vi "nanocal -- nuclear schottky fit -- 2x2 -- V9.vi"() -> ()   [LabVIEW 2021] (continued)
1\" -> 0.000000000000   ,  \"mm2\" -> 0.000000000000   ,  \"mm3\" -> 0.000000000000   ,  \"T\" -> 1.120000000000   ,  \"B\" -> 2.000000000000   ,  \"θ\" -> 90.000000000000   ,  \"Reoff\" -> 0.000000000000   ,  \"Imoff\" -> 0.000000000000   ,  \"στ1\" -> 0.000000000000   ,  \"στS\" -> 0.000000000000   ,  \"στN\" -> 0.000000000000    |>   , \n\"IDS0590_220608_RAW_cal__ref_\" ->   <|    \"ζ\" -> 0.017825574653   ,  \"τ1\" -> 0.116468007826   ,  \"τS\" -> 0.043141778106   ,  \"τN\" -> 0.000373800852   ,  \"τC\" -> 0.002722368928   ,  \"κ0\" -> 0.000000010436   ,  \"mm1\" -> 0.000044937841   ,  \"mm2\" -> 0.046336871767   ,  \"mm3\" -> 0.117099836305   ,  \"T\" -> 1.600000000000   ,  \"B\" -> 2.000000000000   ,  \"θ\" -> 90.000000000000   ,  \"Reoff\" -> -510204.081632653076   ,  \"Imoff\" -> 0.000000000000   ,  \"στ1\" -> 0.011139723010   ,  \"στS\" -> 0.000337999811   ,  \"στN\" -> 0.000011692762    |>   , \n\"IDS0590_220608_RAW_cal__sam_\" ->   <|    \"ζ\" -> 0.000000000000   ,  \"τ1\" -> 0.000000000000   ,  \"τS\" -> 0.000000000000   ,  \"τN\" -> 0.000000000000   ,  \"τC\" -> 0.000000000000   ,  \"κ0\" -> 0.000000000000   ,  \"mm1\" -> 0.000000000000   ,  \"mm2\" -> 0.000000000000   ,  \"mm3\" -> 0.000000000000   ,  \"T\" -> 1.600000000000   ,  \"B\" -> 2.000000000000   ,  \"θ\" -> 90.000000000000   ,  \"Reoff\" -> 0.000000000000   ,  \"Imoff\" -> 0.000000000000   ,  \"στ1\" -> 0.000000000000   ,  \"στS\" -> 0.000000000000   ,  \"στN\" -> 0.000000000000    |>   , \n\"IDS0591_220608_RAW_cal__ref_\" ->   <|    \"ζ\" -> 0.018966449660   ,  \"τ1\" -> 0.110092167291   ,  \"τS\" -> 0.012256930668   ,  \"τN\" -> 0.000242942358   ,  \"τC\" -> 0.002442548821   ,  \"κ0\" -> 0.000000015655   ,  \"mm1\" -> 0.000038124511   ,  \"mm2\" -> 0.014855231202   ,  \"mm3\" -> 0.110378311637   ,  \"T\" -> 2.300000000000   ,  \"B\" -> 2.000000000000   ,  \"θ\" -> 90.000000000000   ,  \"Reoff\" -> -330612.244897959171   ,  \"Imoff\" -> 0.000000000000   ,  \"στ1\" -> 0.010082943855   ,  \"στS\" -> 0.000135571063   ,  \"στN\" -> 0.000004812408    |>   , \n\"IDS0591_220608_RAW_cal__sam_\" ->   <|    \"ζ\" -> 0.000000000000   ,  \"τ1\" -> 0.000000000000   ,  \"τS\" -> 0.000000000000   ,  \"τN\" -> 0.000000000000   ,  \"τC\" -> 0.000000000000   ,  \"κ0\" -> 0.000000000000   ,  \"mm1\" -> 0.000000000000   ,  \"mm2\" -> 0.000000000000   ,  \"mm3\" -> 0.000000000000   ,  \"T\" -> 2.300000000000   ,  \"B\" -> 2.000000000000   ,  \"θ\" -> 90.000000000000   ,  \"Reoff\" -> 0.000000000000   ,  \"Imoff\" -> 0.000000000000   ,  \"στ1\" -> 0.000000000000   ,  \"στS\" -> 0.000000000000   ,  \"στN\" -> 0.000000000000    |>   , \n\"IDS0592_220608_RAW_cal__ref_\" ->   <|    \"ζ\" -> 0.019357316755   ,  \"τ1\" -> 0.109232590741   ,  \"τS\" -> 0.009736709939   ,  \"τN\" -> 0.000148850192   ,  \"τC\" -> 0.002349823712   ,  \"κ0\" -> 0.000000022430   ,  \"mm1\" -> 0.000036187001   ,  \"mm2\" -> 0.012219724348   ,  \"mm3\" -> 0.109403421154   ,  \"T\" -> 3.100000000000   ,  \"B\" -> 2.000000000000   ,  \"θ\" -> 90.000000000000   ,  \"Reoff\" -> -232653.061224489822   ,  \"Imoff\" -> 0.000000000000   ,  \"στ1\" -> 0.008987310328   ,  \"στS\" -> 0.000109754464   ,  \"στN\" -> 0.000004448461    |>   , \n\"IDS0592_220608_RAW_cal__sam_\" ->   <|    \"ζ\" -> 0.000000000000   ,  \"τ1\" -> 0.000000000000   ,  \"τS\" -> 0.000000000000   ,  \"τN\" -> 0.000000000000   ,  \"τC\" -> 0.000000000000   ,  \"κ0\" -> 0.000000000000   ,  \"mm1\" -> 0.000000000000   ,  \"mm2\" -> 0.000000000000   ,  \"mm3\" -> 0.000000000000   ,  \"T\" -> 3.100000000000   ,  \"B\" -> 2.000000000000   ,  \"θ\" -> 90.000000000000   ,  \"Reoff\" -> 0.000000000000   ,  \"Imoff\" -> 0.000000000000   ,  \"στ1\" -> 0.000000000000   ,  \"στS\" -> 0.000000000000   ,  \"στN\" -> 0.000000000000    |>   , \n\"IDS0593_220608_RAW_cal__ref_\" ->   <|    \"ζ\" -> 0.022440001502   ,  \"τ1\" -> 0.108774382212   ,  \"τS\" -> 0.005986162529   ,  \"τN\" -> 0.000081229667   ,  \"τC\" -> 0.001771054543   ,  \"κ0\" -> 0.000000055356   ,  \"mm1\" -> 0.000030262826   ,  \"mm2\" -> 0.007854826642   ,  \"mm3\" -> 0.108863891772   ,  \"T\" -> 5.700000000000   ,  \"B\" -> 2.000000000000   ,  \"θ\" -> 90.000000000000   ,  \"Reoff\" -> -118367.346938775503   ,  \"Imoff\" -> 0.000000000000   ,  \"στ1\" -> 0.009498599420   ,  \"στS\" -> 0.000059156113   ,  \"στN\" -> 0.000001864029    |>   , \n\"IDS0593_220608_RAW_cal__sam_\" ->   <|    \"ζ\" -> 0.000000000000   ,  \"τ1\" -> 0.000000000000   ,  \"τS\" -> 0.000000000000   ,  \"τN\" -> 0.000000000000   ,  \"τC\" -> 0.000000000000   ,  \"κ0\" -> 0.000000000000   ,  \"mm1\" -> 0.000000000000   ,  \"mm2\" -> 0.000000000000   ,  \"mm3\" -> 0.000000000000   ,  \"T\" -> 5.700000000000   ,  \"B\" -> 2.000000000000   ,  \"θ\" -> 90.000000000000   ,  \"Reoff\" -> 0.000000000000   ,  \"Imoff\" -> 0.000000000000   ,  \"στ1\" -> 0.000000000000   ,  \"στS\" -> 0.000000000000   ,  \"στN\" -> 0.000000000000    |>   , \n\"IDS0595_220608_RAW_cal__ref_\" ->   <|    \"ζ\" -> 0.258873400405   ,  \"τ1\" -> 0.044703065528   ,  \"τS\" -> 0.045959272173   ,  \"τN\" -> 0.010257269472   ,  \"τC\" -> 0.000790030370   ,  \"κ0\" -> 0.000000000876   ,  \"mm1\" -> 0.000160711520   ,  \"mm2\" -> 0.030566838015   ,  \"mm3\" -> 0.085535055303   ,  \"T\" -> 0.200000000000   ,  \"B\" -> 4.000000000000   ,  \"θ\" -> 90.000000000000   ,  \"Reoff\" -> -50122448.979591846500   ,  \"Imoff\" -> 0.000000000000   ,  \"στ1\" -> 0.022832091218   ,  \"στS\" -> 0.001836443517   ,  \"στN\" -> 0.003113362841    |>   , \n\"IDS0595_220608_RAW_cal__sam_\" ->   <|    \"ζ\" -> 0.000000000000   ,  \"τ1\" -> 0.000000000000   ,  \"τS\" -> 0.000000000000   ,  \"τN\" -> 0.000000000000   ,  \"τC\" -> 0.000000000000   ,  \"κ0\" -> 0.000000000000   ,  \"mm1\" -> 0.000000000000   ,  \"mm2\" -> 0.000000000000   ,  \"mm3\" -> 0.000000000000   ,  \"T\" -> 0.200000000000   ,  \"B\" -> 4.000000000000   ,  \"θ\" -> 90.000000000000   ,  \"Reoff\" -> 0.000000000000   ,  \"Imoff\" -> 0.000000000000   ,  \"στ1\" -> 0.000000000000   ,  \"στS\" -> 0.000000000000   ,  \"στN\" -> 0.000000000000    |>   , \n\"IDS0596_220608_RAW_cal__ref_\" ->   <|    \"ζ\" -> 0.360293553844   ,  \"τ1\" -> 0.054491247205   ,  \"τS\" -> 0.052365925569   ,  \"τN\" -> 0.021163604976   ,  \"τC\" -> 0.000735569124   ,  \"κ0\" -> 0.000000000708   ,  \"mm1\" -> 0.000193352298   ,  \"mm2\" -> 0.031708785760   ,  \"mm3\" -> 0.123346424689   ,  \"T\" -> 0.170000000000   ,  \"B\" -> 4.000000000000   ,  \"θ\" -> 90.000000000000   ,  \"Reoff\" -> -91020408.163265347500   ,  \"Imoff\" -> 0.000000000000   ,  \"στ1\" -> 0.039757626567   ,  \"στS\" -> 0.004569334706   ,  \"στN\" -> 0.007867287880    |>   , \n\"IDS0596_220608_RAW_cal__sam_\" ->   <|    \"ζ\" -> 0.000000000000   ,  \"τ1\" -> 0.000000000000   ,  \"τS\" -> 0.000000000000   ,  \"τN\" -> 0.000000000000   ,  \"τC\" -> 0.000000000000   ,  \"κ0\" -> 0.000000000000   ,  \"mm1\" -> 0.000000000000   ,  \"mm2\" -> 0.000000000000   ,  \"mm3\" -> 0.000000000000   ,  \"T\" -> 0.170000000000   ,  \"B\" -> 4.000000000000   ,  \"θ\" -> 90.000000000000   ,  \"Reoff\" -> 0.000000000000   ,  \"Imoff\" -> 0.000000000000   ,  \"στ1\" -> 0.000000000000   ,  \"στS\" -> 0.000000000000   ,  \"στN\" -> 0.000000000000    |>   , \n\"IDS0597_220608_RAW_cal__ref_\" ->   <|    \"ζ\" -> 0.463165977160   ,  \"τ1\" -> 0.056305688672   ,  \"τS\" -> 0.058936067293   ,  \"τN\" -> 0.032266294348   ,  \"τC\" -> 0.000690215533   ,  \"κ0\" -> 0.000000000590   ,  \"mm1\" -> 0.000217293879   ,  \"mm2\" -> 0.030581784486   ,  \"mm3\" -> 0.159641018430   ,  \"T\" -> 0.150000000000   ,  \"B\" -> 4.000000000000   ,  \"θ\" -> 90.000000000000   ,  \"Reoff\" -> -129873469.387755096000   ,  \"Imoff\" -> 0.000000000000   ,  \"στ1\" -> 0.023207253822   ,  \"στS\" -> 0.004087293472   ,  \"στN\" -> 0.007020371426    |>   , \n\"IDS0597_220608_RAW_cal__sam_\" ->   <|    \"ζ\" -> 0.000000000000   ,  \"τ1\" -> 0.000000000000   ,  \"τS\" -> 0.000000000000   ,  \"τN\" -> 0.000000000000   ,  \"τC\" -> 0.000000000000   ,  \"κ0\" -> 0.000000000000   ,  \"mm1\" -> 0.000000000000   ,  \"mm2\" -> 0.000000000000   ,  \"mm3\" -> 0.000000000000   ,  \"T\" -> 0.150000000000   ,  \"B\" -> 4.000000000000   ,  \"θ\" -> 90.000000000000   ,  \"Reoff\" -> 0.000000000000   ,  \"Imoff\" -> 0.000000000000   ,  \"στ1\" -> 0.000000000000   ,  \"στS\" -> 0.000000000000   ,  \"στN\" -> 0.000000000000    |>   , \n\"IDS0598_220609_RAW_cal__ref_\" ->   <|    \"ζ\" -> 0.667698633058   ,  \"τ1\" -> 0.058414013789   ,  \"τS\" -> 0.079345994200   ,  \"τN\" -> 0.070623883647   ,  \"τC\" -> 0.000796244293   ,  \"κ0\" -> 0.000000000447   ,  \"mm1\" -> 0.000317638863   ,  \"mm2\" -> 0.027565245662   ,  \"mm3\" -> 0.281431933842   ,  \"T\" -> 0.120000000000   ,  \"B\" -> 4.000000000000   ,  \"θ\" -> 90.000000000000   ,  \"Reoff\" -> -199400000.000000000000   ,  \"Imoff\" -> 0.000000000000   ,  \"στ1\" -> 0.061256230703   ,  \"στS\" -> 0.021100595545   ,  \"στN\" -> 0.037759623008    |>   , \n\"IDS0598_220609_RAW_cal__sam_\" ->   <|    \"ζ\" -> 0.000000000000   ,  \"τ1\" -> 0.000000000000   ,  \"τS\" -> 0.000000000000   ,  \"τN\" -> 0.000000000000   ,  \"τC\" -> 0.000000000000   ,  \"κ0\" -> 0.000000000000   ,  \"mm1\" -> 0.000000000000   ,  \"mm2\" -> 0.000000000000   ,  \"mm3\" -> 0.000000000000   ,  \"T\" -> 0.120000000000   ,  \"B\" -> 4.000000000000   ,  \"θ\" -> 90.000000000000   ,  \"Reoff\" -> 0.000000000000   ,  \"Imoff\" -> 0.000000000000   ,  \"στ1\" -> 0.000000000000   ,  \"στS\" -> 0.000000000000   ,  \"στN\" -> 0.000000000000    |>   , \n\"IDS0599_220609_RAW_cal__ref_\" ->   <|    \"ζ\" -> 0.172195485890   ,  \"τ1\" -> 0.041384778581   ,  \"τS\" -> 0.038526635798   ,  \"τN\" -> 0.004361184391   ,  \"τC\" -> 0.000785294253   ,  \"κ0\" -> 0.000000001211   ,  \"mm1\" -> 0.000113668710   ,  \"mm2\" -> 0.030854392047   ,  \"mm3\" -> 0.061474921303   ,  \"T\" -> 0.250000000000   ,  \"B\" -> 4.000000000000   ,  \"θ\" -> 90.000000000000   ,  \"Reoff\" -> -31567346.938775509600   ,  \"Imoff\" -> 0.000000000000   ,  \"στ1\" -> 0.007771542596   ,  \"στS\" -> 0.000527239898   ,  \"στN\" -> 0.000989287072    |>   , \n\"IDS0599_220609_RAW_cal__sam_\" ->   <|    \"ζ\" -> 0.000000000000   ,  \"τ1\" -> 0.000000000000   ,  \"τS\" -> 0.000000000000   ,  \"τN\" -> 0.000000000000   ,  \"τC\" -> 0.000000000000   ,  \"κ0\" -> 0.000000000000   ,  \"mm1\" -> 0.000000000000   ,  \"mm2\" -> 0.000000000000   ,  \"mm3\" -> 0.000000000000   ,  \"T\" -> 0.250000000000   ,  \"B\" -> 4.000000000000   ,  \"θ\" -> 90.000000000000   ,  \"Reoff\" -> 0.000000000000   ,  \"Imoff\" -> 0.000000000000   ,  \"στ1\" -> 0.000000000000   ,  \"στS\" -> 0.000000000000   ,  \"στN\" -> 0.000000000000    |>   , \n\"IDS0601_220609_RAW_cal__ref_\" ->   <|    \"ζ\" -> 0.088588946696   ,  \"τ1\" -> 0.041065464736   ,  \"τS\" -> 0.032932718499   ,  \"τN\" -> 0.001668080480   ,  \"τC\" -> 0.000981218773   ,  \"κ0\" -> 0.000000001942   ,  \"mm1\" -> 0.000077888432   ,  \"mm2\" -> 0.031092575692   ,  \"mm3\" -> 0.048542266701   ,  \"T\" -> 0.360000000000   ,  \"B\" -> 4.000000000000   ,  \"θ\" -> 90.000000000000   ,  \"Reoff\" -> -11367346.938775509600   ,  \"Imoff\" -> 0.000000000000   ,  \"στ1\" -> 0.003759438303   ,  \"στS\" -> 0.000267670309   ,  \"στN\" -> 0.000061047491    |>   , \n\"IDS0601_220609_RAW_cal__sam_\" ->   <|    \"ζ\" -> 0.000000000000   ,  \"τ1\" -> 0.000000000000   ,  \"τS\" -> 0.000000000000   ,  \"τN\" -> 0.000000000000   ,  \"τC\" -> 0.000000000000   ,  \"κ0\" -> 0.000000000000   ,  \"mm1\" -> 0.000000000000   ,  \"mm2\" -> 0.000000000000   ,  \"mm3\" -> 0.000000000000   ,  \"T\" -> 0.360000000000   ,  \"B\" -> 4.000000000000   ,  \"θ\" -> 90.000000000000   ,  \"Reoff\" -> 0.000000000000   ,  \"Imoff\" -> 0.000000000000   ,  \"στ1\" -> 0.000000000000   ,  \"στS\" -> 0.000000000000   ,  \"στN\" -> 0.000000000000    |>   , \n\"IDS0602_220609_RAW_cal__ref_\" ->   <|    \"ζ\" -> 0.070839718876   ,  \"τ1\" -> 0.038371041474   ,  \"τS\" -> 0.031637984426   ,  \"τN\" -> 0.001186889357   ,  \"τC\" -> 0.001025755146   ,  \"κ0\" -> 0.000000002344   ,  \"mm1\" -> 0.000065987726   ,  \"mm2\" -> 0.030166305884   ,  \"mm3\" -> 0.044314681623   ,  \"T\" -> 0.420000000000   ,  \"B\" -> 4.000000000000   ,  \"θ\" -> 90.000000000000   ,  \"Reoff\" -> -8473469.387755101550   ,  \"Imoff\" -> 0.000000000000   ,  \"στ1\" -> 0.001572734023   ,  \"στS\" -> 0.000244025601   ,  \"στN\" -> 0.000010717849    |>   , \n\"IDS0602_220609_RAW_cal__sam_\" ->   <|    \"ζ\" -> 0.000000000000   ,  \"τ1\" -> 0.000000000000   ,  \"τS\" -> 0.000000000000   ,  \"τN\" -> 0.000000000000   ,  \"τC\" -> 0.000000000000   ,  \"κ0\" -> 0.000000000000   ,  \"mm1\" -> 0.000000000000   ,  \"mm2\" -> 0.000000000000   ,  \"mm3\" -> 0.000000000000   ,  \"T\" -> 0.420000000000   ,  \"B\" -> 4.000000000000   ,  \"θ\" -> 90.000000000000   ,  \"Reoff\" -> 0.000000000000   ,  \"Imoff\" -> 0.000000000000   ,  \"στ1\" -> 0.000000000000   ,  \"στS\" -> 0.000000000000   ,  \"στN\" -> 0.000000000000    |>   , \n\"IDS0603_220609_RAW_cal__ref_\" ->   <|    \"ζ\" -> 0.046492492626   ,  \"τ1\" -> 0.038232445790   ,  \"τS\" -> 0.031093656328   ,  \"τN\" -> 0.000672520001   ,  \"τC\" -> 0.001537595786   ,  \"κ0\" -> 0.000000003028   ,  \"mm1\" -> 0.000065353683   ,  \"mm2\" -> 0.030996834866   ,  \"mm3\" -> 0.041950918075   ,  \"T\" -> 0.520000000000   ,  \"B\" -> 4.000000000000   ,  \"θ\" -> 90.000000000000   ,  \"Reoff\" -> -3085714.285714285450   ,  \"Imoff\" -> 0.000000000000   ,  \"στ1\" -> 0.001914222591   ,  \"στS\" -> 0.000173880223   ,  \"στN\" -> 0.000009749430    |>   , \n\"IDS0603_220609_RAW_cal__sam_\" ->   <|    \"ζ\" -> 0.000000000000   ,  \"τ1\" -> 0.000000000000   ,  \"τS\" -> 0.000000000000   ,  \"τN\" -> 0.000000000000   ,  \"τC\" -> 0.000000000000   ,  \"κ0\" -> 0.000000000000   ,  \"mm1\" -> 0.000000000000   ,  \"mm2\" -> 0.000000000000   ,  \"mm3\" -> 0.000000000000   ,  \"T\" -> 0.520000000000   ,  \"B\" -> 4.000000000000   ,  \"θ\" -> 90.000000000000   ,  \"Reoff\" -> 0.000000000000   ,  \"Imoff\" -> 0.000000000000   ,  \"στ1\" -> 0.000000000000   ,  \"στS\" -> 0.000000000000   ,  \"στN\" -> 0.000000000000    |>   , \n\"IDS0604_220609_RAW_cal__ref_\" ->   <|    \"ζ\" -> 0.038076441388   ,  \"τ1\" -> 0.037827631760   ,  \"τS\" -> 0.031677046924   ,  \"τN\" -> 0.000456015371   ,  \"τC\" -> 0.001552950065   ,  \"κ0\" -> 0.000000003729   ,  \"mm1\" -> 0.000054479261   ,  \"mm2\" -> 0.031856398472   ,  \"mm3\" -> 0.040826279050   ,  \"T\" -> 0.620000000000   ,  \"B\" -> 4.000000000000   ,  \"θ\" -> 90.000000000000   ,  \"Reoff\" -> -2502040.816326530650   ,  \"Imoff\" -> 0.000000000000   ,  \"στ1\" -> 0.001808471812   ,  \"στS\" -> 0.000207619665   ,  \"στN\" -> 0.000014710860    |>   , \n\"IDS0604_220609_RAW_cal__sam_\" ->   <|    \"ζ\" -> 0.000000000000   ,  \"τ1\" -> 0.000000000000   ,  \"τS\" -> 0.000000000000   ,  \"τN\" -> 0.000000000000   ,  \"τC\" -> 0.000000000000   ,  \"κ0\" -> 0.000000000000   ,  \"mm1\" -> 0.000000000000   ,  \"mm2\" -> 0.000000000000   ,  \"mm3\" -> 0.000000000000   ,  \"T\" -> 0.620000000000   ,  \"B\" -> 4.000000000000   ,  \"θ\" -> 90.000000000000   ,  \"Reoff\" -> 0.000000000000   ,  \"Imoff\" -> 0.000000000000   ,  \"στ1\" -> 0.000000000000   ,  \"στS\" -> 0.000000000000   ,  \"στN\" -> 0.000000000000    |>   , \n\"IDS0605_220609_RAW_cal__ref_\" ->   <|    \"ζ\" -> 0.029084199331   ,  \"τ1\" -> 0.037802339111   ,  \"τS\" -> 0.034441444992   ,  \"τN\" -> 0.000221453940   ,  \"τC\" -> 0.001674221350   ,  \"κ0\" -> 0.000000005054   ,  \"mm1\" -> 0.000045238028   ,  \"mm2\" -> 0.034605412143   ,  \"mm3\" -> 0.040496951884   ,  \"T\" -> 0.820000000000   ,  \"B\" -> 4.000000000000   ,  \"θ\" -> 90.000000000000   ,  \"Reoff\" -> -1648979.591836734680   ,  \"Imoff\" -> 0.000000000000   ,  \"στ1\" -> 0.004366885644   ,  \"στS\" -> 0.000226589736   ,  \"στN\" -> 0.000007619141    |>   , \n\"IDS0605_220609_RAW_cal__sam_\" ->   <|    \"ζ\" -> 0.000000000000   ,  \"τ1\" -> 0.000000000000   ,  \"τS\" -> 0.000000000000   ,  \"τN\" -> 0.000000000000   ,  \"τC\" -> 0.000000000000   ,  \"κ0\" -> 0.000000000000   ,  \"mm1\" -> 0.000000000000   ,  \"mm2\" -> 0.000000000000   ,  \"mm3\" -> 0.000000000000   ,  \"T\" -> 0.820000000000   ,  \"B\" -> 4.000000000000   ,  \"θ\" -> 90.000000000000   ,  \"Reoff\" -> 0.000000000000   ,  \"Imoff\" -> 0.000000000000   ,  \"στ1\" -> 0.000000000000   ,  \"στS\" -> 0.000000000000   ,  \"στN\" -> 0.000000000000    |>   , \n\"IDS0606_220609_RAW_cal__ref_\" ->   <|    \"ζ\" -> 0.021888227668   ,  \"τ1\" -> 0.037829739612   ,  \"τS\" -> 0.039149374988   ,  \"τN\" -> 0.000098261842   ,  \"τC\" -> 0.001756976577   ,  \"κ0\" -> 0.000000007009   ,  \"mm1\" -> 0.000036081312   ,  \"mm2\" -> 0.037036868509   ,  \"mm3\" -> 0.042620464409   ,  \"T\" -> 1.100000000000   ,  \"B\" -> 4.000000000000   ,  \"θ\" -> 90.000000000000   ,  \"Reoff\" -> -840816.326530613004   ,  \"Imoff\" -> 0.000000000000   ,  \"στ1\" -> 0.002337246267   ,  \"στS\" -> 0.000239648135   ,  \"στN\" -> 0.000002696186    |>   , \n\"IDS0606_220609_RAW_cal__sam_\" ->   <|    \"ζ\" -> 0.000000000000   ,  \"τ1\" -> 0.000000000000   ,  \"τS\" -> 0.000000000000   ,  \"τN\" -> 0.000000000000   ,  \"τC\" -> 0.000000000000   ,  \"κ0\" -> 0.000000000000   ,  \"mm1\" -> 0.000000000000   ,  \"mm2\" -> 0.000000000000   ,  \"mm3\" -> 0.000000000000   ,  \"T\" -> 1.100000000000   ,  \"B\" -> 4.000000000000   ,  \"θ\" -> 90.000000000000   ,  \"Reoff\" -> 0.000000000000   ,  \"Imoff\" -> 0.000000000000   ,  \"στ1\" -> 0.000000000000   ,  \"στS\" -> 0.000000000000   ,  \"στN\" -> 0.000000000000    |>   , \n\"IDS0607_220609_RAW_cal__ref_\" ->   <|    \"ζ\" -> 0.018621761780   ,  \"τ1\" -> 0.037381709477   ,  \"τS\" -> 0.015442772270   ,  \"τN\" -> 0.000037477448   ,  \"τC\" -> 0.001928945161   ,  \"κ0\" -> 0.000000010412   ,  \"mm1\" -> 0.000031467858   ,  \"mm2\" -> 0.017593885804   ,  \"mm3\" -> 0.037453820216   ,  \"T\" -> 1.600000000000   ,  \"B\" -> 4.000000000000   ,  \"θ\" -> 90.000000000000   ,  \"Reoff\" -> -583673.469387755030   ,  \"Imoff\" -> 0.000000000000   ,  \"στ1\" -> 0.004296807814   ,  \"στS\" -> 0.000140639084   ,  \"στN\" -> 0.000001749476    |>   , \n\"IDS0607_220609_RAW_cal__sam_\" ->   <|    \"ζ\" -> 0.000000000000   ,  \"τ1\" -> 0.000000000000   ,  \"τS\" -> 0.000000000000   ,  \"τN\" -> 0.000000000000   ,  \"τC\" -> 0.000000000000   ,  \"κ0\" -> 0.000000000000   ,  \"mm1\" -> 0.000000000000   ,  \"mm2\" -> 0.000000000000   ,  \"mm3\" -> 0.000000000000   ,  \"T\" -> 1.600000000000   ,  \"B\" -> 4.000000000000   ,  \"θ\" -> 90.000000000000   ,  \"Reoff\" -> 0.000000000000   ,  \"Imoff\" -> 0.000000000000   ,  \"στ1\" -> 0.000000000000   ,  \"στS\" -> 0.000000000000   ,  \"στN\" -> 0.000000000000    |>   , \n\"IDS0608_220610_RAW_cal__ref_\" ->   <|    \"ζ\" -> 0.016544796602   ,  \"τ1\" -> 0.037383789571   ,  \"τS\" -> 0.013791768179   ,  \"τN\" -> 0.000022452051   ,  \"τC\" -> 0.002003011160   ,  \"κ0\" -> 0.000000012629   ,  \"mm1\" -> 0.000028575716   ,  \"mm2\" -> 0.015977354879   ,  \"mm3\" -> 0.037423643830   ,  \"T\" -> 1.900000000000   ,  \"B\" -> 4.000000000000   ,  \"θ\" -> 90.000000000000   ,  \"Reoff\" -> -306122.448979591834   ,  \"Imoff\" -> 0.000000000000   ,  \"στ1\" -> 0.018453773805   ,  \"στS\" -> 0.003656712594   ,  \"στN\" -> 0.000009862061    |>   , \n\"IDS0608_220610_RAW_cal__sam_\" ->   <|    \"ζ\" -> 0.000000000000   ,  \"τ1\" -> 0.000000000000   ,  \"τS\" -> 0.000000000000   ,  \"τN\" -> 0.000000000000   ,  \"τC\" -> 0.000000000000   ,  \"κ0\" -> 0.000000000000   ,  \"mm1\" -> 0.000000000000   ,  \"mm2\" -> 0.000000000000   ,  \"mm3\" -> 0.000000000000   ,  \"T\" -> 1.900000000000   ,  \"B\" -> 4.000000000000   ,  \"θ\" -> 90.000000000000   ,  \"Reoff\" -> 0.000000000000   ,  \"Imoff\" -> 0.000000000000   ,  \"στ1\" -> 0.000000000000   ,  \"στS\" -> 0.000000000000   ,  \"στN\" -> 0.000000000000    |>   , \n\"IDS0609_220610_RAW_cal__ref_\" ->   <|    \"ζ\" -> 0.016105107000   ,  \"τ1\" -> 0.037302695889   ,  \"τS\" -> 0.009839075109   ,  \"τN\" -> 0.000006613992   ,  \"τC\" -> 0.002285007383   ,  \"κ0\" -> 0.000000022392   ,  \"mm1\" -> 0.000029550397   ,  \"mm2\" -> 0.012249707235   ,  \"mm3\" -> 0.037312700617   ,  \"T\" -> 3.100000000000   ,  \"B\" -> 4.000000000000   ,  \"θ\" -> 90.000000000000   ,  \"Reoff\" -> -175510.204081632662   ,  \"Imoff\" -> 0.000000000000   ,  \"στ1\" -> 0.000595847504   ,  \"στS\" -> 0.000046124245   ,  \"στN\" -> 0.000000091796    |>   , \n\"IDS0609_220610_RAW_cal__sam_\" ->   <|    \"ζ\" -> 0.000000000000   ,  \"τ1\" -> 0.000000000000   ,  \"τS\" -> 0.000000000000   ,  \"τN\" -> 0.000000000000   ,  \"τC\" -> 0.000000000000   ,  \"κ0\" -> 0.000000000000   ,  \"mm1\" -> 0.000000000000   ,  \"mm2\" -> 0.000000000000   ,  \"mm3\" -> 0.000000000000   ,  \"T\" -> 3.100000000000   ,  \"B\" -> 4.000000000000   ,  \"θ\" -> 90.000000000000   ,  \"Reoff\" -> 0.000000000000   ,  \"Imoff\" -> 0.000000000000   ,  \"στ1\" -> 0.000000000000   ,  \"στS\" -> 0.000000000000   ,  \"στN\" -> 0.000000000000    |>   , \n\"IDS0610_220610_RAW_cal__ref_\" ->   <|    \"ζ\" -> 0.017289416692   ,  \"τ1\" -> 0.037297104830   ,  \"τS\" -> 0.006044321671   ,  \"τN\" -> 0.000001504072   ,  \"τC\" -> 0.001946264025   ,  \"κ0\" -> 0.000000055145   ,  \"mm1\" -> 0.000025203584   ,  \"mm2\" -> 0.008069462881   ,  \"mm3\" -> 0.037299056933   ,  \"T\" -> 5.700000000000   ,  \"B\" -> 4.000000000000   ,  \"θ\" -> 90.000000000000   ,  \"Reoff\" -> -61224.489795918343   ,  \"Imoff\" -> 0.000000000000   ,  \"στ1\" -> 0.009662236305   ,  \"στS\" -> 0.002526126048   ,  \"στN\" -> 0.000001649991    |>   , \n\"IDS0610_220610_RAW_cal__sam_\" ->   <|    \"ζ\" -> 0.000000000000   ,  \"τ1\" -> 0.000000000000   ,  \"τS\" -> 0.000000000000   ,  \"τN\" -> 0.000000000000   ,  \"τC\" -> 0.000000000000   ,  \"κ0\" -> 0.000000000000   ,  \"mm1\" -> 0.000000000000   ,  \"mm2\" -> 0.000000000000   ,  \"mm3\" -> 0.000000000000   ,  \"T\" -> 5.700000000000   ,  \"B\" -> 4.000000000000   ,  \"θ\" -> 90.000000000000   ,  \"Reoff\" -> 0.000000000000   ,  \"Imoff\" -> 0.000000000000   ,  \"στ1\" -> 0.000000000000   ,  \"στS\" -> 0.000000000000   ,  \"στN\" -> 0.000000000000    |>   , \n\"IDS0612_220610_RAW_cal__ref_\" ->   <|    \"ζ\" -> 0.027806171987   ,  \"τ1\" -> 0.017638558844   ,  \"τS\" -> 0.022454693159   ,  \"τN\" -> 0.000230606872   ,  \"τC\" -> 0.002790453039   ,  \"κ0\" -> 0.000000005094   ,  \"mm1\" -> 0.000067525510   ,  \"mm2\" -> 0.017167524250   ,  \"mm3\" -> 0.026510053509   ,  \"T\" -> 0.820000000000   ,  \"B\" -> 5.000000000000   ,  \"θ\" -> 90.000000000000   ,  \"Reoff\" -> -885714.285714285680   ,  \"Imoff\" -> 0.000000000000   ,  \"στ1\" -> 0.001146653541   ,  \"στS\" -> 0.000179915023   ,  \"στN\" -> 0.000004482288    |>   , \n\"IDS0612_220610_RAW_cal__sam_\" ->   <|    \"ζ\" -> 0.000000000000   ,  \"τ1\" -> 0.000000000000   ,  \"τS\" -> 0.000000000000   ,  \"τN\" -> 0.000000000000   ,  \"τC\" -> 0.000000000000   ,  \"κ0\" -> 0.000000000000   ,  \"mm1\" -> 0.000000000000   ,  \"mm2\" -> 0.000000000000   ,  \"mm3\" -> 0.000000000000   ,  \"T\" -> 0.820000000000   ,  \"B\" -> 5.000000000000   ,  \"θ\" -> 90.000000000000   ,  \"Reoff\" -> 0.000000000000   ,  \"Imoff\" -> 0.000000000000   ,  \"στ1\" -> 0.000000000000   ,  \"στS\" -> 0.000000000000   ,  \"στN\" -> 0.000000000000    |>   , \n\"IDS0613_220610_RAW_cal__ref_\" ->   <|    \"ζ\" -> 0.023917075048   ,  \"τ1\" -> 0.017613265802   ,  \"τS\" -> 0.018183300032   ,  \"τN\" -> 0.000148874581   ,  \"τC\" -> 0.002629507092   ,  \"κ0\" -> 0.000000007146   ,  \"mm1\" -> 0.000053956796   ,  \"mm2\" -> 0.016996296873   ,  \"mm3\" -> 0.021963145834   ,  \"T\" -> 1.120000000000   ,  \"B\" -> 5.000000000000   ,  \"θ\" -> 90.000000000000   ,  \"Reoff\" -> -877551.020408163311   ,  \"Imoff\" -> 0.000000000000   ,  \"στ1\" -> 0.001189746119   ,  \"στS\" -> 0.000158276904   ,  \"στN\" -> 0.000002453686    |>   , \n\"IDS0613_220610_RAW_cal__sam_\" ->   <|    \"ζ\" -> 0.000000000000   ,  \"τ1\" -> 0.000000000000   ,  \"τS\" -> 0.000000000000   ,  \"τN\" -> 0.000000000000   ,  \"τC\" -> 0.000000000000   ,  \"κ0\" -> 0.000000000000   ,  \"mm1\" -> 0.000000000000   ,  \"mm2\" -> 0.000000000000   ,  \"mm3\" -> 0.000000000000   ,  \"T\" -> 1.120000000000   ,  \"B\" -> 5.000000000000   ,  \"θ\" -> 90.000000000000   ,  \"Reoff\" -> 0.000000000000   ,  \"Imoff\" -> 0.000000000000   ,  \"στ1\" -> 0.000000000000   ,  \"στS\" -> 0.000000000000   ,  \"στN\" -> 0.000000000000    |>   , \n\"IDS0614_220610_RAW_cal__ref_\" ->   <|    \"ζ\" -> 0.017909358082   ,  \"τ1\" -> 0.017480687226   ,  \"τS\" -> 0.012860329043   ,  \"τN\" -> 0.000077799463   ,  \"τC\" -> 0.003015067786   ,  \"κ0\" -> 0.000000012573   ,  \"mm1\" -> 0.000043232989   ,  \"mm2\" -> 0.015457741040   ,  \"mm3\" -> 0.018164623065   ,  \"T\" -> 1.900000000000   ,  \"B\" -> 5.000000000000   ,  \"θ\" -> 90.000000000000   ,  \"Reoff\" -> -330612.244897959171   ,  \"Imoff\" -> 0.000000000000   ,  \"στ1\" -> 0.000912905894   ,  \"στS\" -> 0.000088716304   ,  \"στN\" -> 0.000002113548    |>   , \n\"IDS0614_220610_RAW_cal__sam_\" ->   <|    \"ζ\" -> 0.000000000000   ,  \"τ1\" -> 0.000000000000   ,  \"τS\" -> 0.000000000000   ,  \"τN\" -> 0.000000000000   ,  \"τC\" -> 0.000000000000   ,  \"κ0\" -> 0.000000000000   ,  \"mm1\" -> 0.000000000000   ,  \"mm2\" -> 0.000000000000   ,  \"mm3\" -> 0.000000000000   ,  \"T\" -> 1.900000000000   ,  \"B\" -> 5.000000000000   ,  \"θ\" -> 90.000000000000   ,  \"Reoff\" -> 0.000000000000   ,  \"Imoff\" -> 0.000000000000   ,  \"στ1\" -> 0.000000000000   ,  \"στS\" -> 0.000000000000   ,  \"στN\" -> 0.000000000000    |>   , \n\"IDS0615_220610_RAW_cal__ref_\" ->   <|    \"ζ\" -> 0.018184973350   ,  \"τ1\" -> 0.017408880913   ,  \"τS\" -> 0.009354983655   ,  \"τN\" -> 0.000026355523   ,  \"τC\" -> 0.002778499813   ,  \"κ0\" -> 0.000000022360   ,  \"mm1\" -> 0.000038538571   ,  \"mm2\" -> 0.012202232609   ,  \"mm3\" -> 0.017498548126   ,  \"T\" -> 3.100000000000   ,  \"B\" -> 5.000000000000   ,  \"θ\" -> 90.000000000000   ,  \"Reoff\" -> -191836.734693877515   ,  \"Imoff\" -> 0.000000000000   ,  \"στ1\" -> 0.001312365409   ,  \"στS\" -> 0.000063057161   ,  \"στN\" -> 0.000000988894    |>   , \n\"IDS0615_220610_RAW_cal__sam_\" ->   <|    \"ζ\" -> 0.000000000000   ,  \"τ1\" -> 0.000000000000   ,  \"τS\" -> 0.000000000000   ,  \"τN\" -> 0.000000000000   ,  \"τC\" -> 0.000000000000   ,  \"κ0\" -> 0.000000000000   ,  \"mm1\" -> 0.000000000000   ,  \"mm2\" -> 0.000000000000   ,  \"mm3\" -> 0.000000000000   ,  \"T\" -> 3.100000000000   ,  \"B\" -> 5.000000000000   ,  \"θ\" -> 90.000000000000   ,  \"Reoff\" -> 0.000000000000   ,  \"Imoff\" -> 0.000000000000   ,  \"στ1\" -> 0.000000000000   ,  \"στS\" -> 0.000000000000   ,  \"στN\" -> 0.000000000000    |>   , \n\"IDS0616_220610_RAW_cal__ref_\" ->   <|    \"ζ\" -> 0.021580744060   ,  \"τ1\" -> 0.018863304594   ,  \"τS\" -> 0.006040479317   ,  \"τN\" -> 0.000014968890   ,  \"τC\" -> 0.001981910818   ,  \"κ0\" -> 0.000000054950   ,  \"mm1\" -> 0.000031813796   ,  \"mm2\" -> 0.008109417181   ,  \"mm3\" -> 0.018890113720   ,  \"T\" -> 5.700000000000   ,  \"B\" -> 5.000000000000   ,  \"θ\" -> 90.000000000000   ,  \"Reoff\" -> -102040.816326530650   ,  \"Imoff\" -> 0.000000000000   ,  \"στ1\" -> 0.003832459400   ,  \"στS\" -> 0.000063285444   ,  \"στN\" -> 0.000001437164    |>   , \n\"IDS0616_220610_RAW_cal__sam_\" ->   <|    \"ζ\" -> 0.000000000000   ,  \"τ1\" -> 0.000000000000   ,  \"τS\" -> 0.000000000000   ,  \"τN\" -> 0.000000000000   ,  \"τC\" -> 0.000000000000   ,  \"κ0\" -> 0.000000000000   ,  \"mm1\" -> 0.000000000000   ,  \"mm2\" -> 0.000000000000   ,  \"mm3\" -> 0.000000000000   ,  \"T\" -> 5.700000000000   ,  \"B\" -> 5.000000000000   ,  \"θ\" -> 90.000000000000   ,  \"Reoff\" -> 0.000000000000   ,  \"Imoff\" -> 0.000000000000   ,  \"στ1\" -> 0.000000000000   ,  \"στS\" -> 0.000000000000   ,  \"στN\" -> 0.000000000000    |>   , \n\"IDS0618_220610_RAW_cal__ref_\" ->   <|    \"ζ\" -> 0.038971550776   ,  \"τ1\" -> 0.018146117143   ,  \"τS\" -> 0.027126639064   ,  \"τN\" -> 0.001095165707   ,  \"τC\" -> 0.001889759396   ,  \"κ0\" -> 0.000000003734   ,  \"mm1\" -> 0.000066576943   ,  \"mm2\" -> 0.016715518022   ,  \"mm3\" -> 0.032575433843   ,  \"T\" -> 0.620000000000   ,  \"B\" -> 8.000000000000   ,  \"θ\" -> 90.000000000000   ,  \"Reoff\" -> -2648979.591836734680   ,  \"Imoff\" -> 0.000000000000   ,  \"στ1\" -> 0.003517417724   ,  \"στS\" -> 0.000462948011   ,  \"στN\" -> 0.000116737620    |>   , \n\"IDS0618_220610_RAW_cal__sam_\" ->   <|    \"ζ\" -> 0.000000000000   ,  \"τ1\" -> 0.000000000000   ,  \"τS\" -> 0.000000000000   ,  \"τN\" -> 0.000000000000   ,  \"τC\" -> 0.000000000000   ,  \"κ0\" -> 0.000000000000   ,  \"mm1\" -> 0.000000000000   ,  \"mm2\" -> 0.000000000000   ,  \"mm3\" -> 0.000000000000   ,  \"T\" -> 0.620000000000   ,  \"B\" -> 8.000000000000   ,  \"θ\" -> 90.000000000000   ,  \"Reoff\" -> 0.000000000000   ,  \"Imoff\" -> 0.000000000000   ,  \"στ1\" -> 0.000000000000   ,  \"στS\" -> 0.000000000000   ,  \"στN\" -> 0.000000000000    |>   , \n\"IDS0619_220610_RAW_cal__ref_\" ->   <|    \"ζ\" -> 0.024009223885   ,  \"τ1\" -> 0.018709750105   ,  \"τS\" -> 0.019196212155   ,  \"τN\" -> 0.000222399775   ,  \"τC\" -> 0.002606828702   ,  \"κ0\" -> 0.000000007177   ,  \"mm1\" -> 0.000054095260   ,  \"mm2\" -> 0.017792742522   ,  \"mm3\" -> 0.023354578757   ,  \"T\" -> 1.120000000000   ,  \"B\" -> 8.000000000000   ,  \"θ\" -> 90.000000000000   ,  \"Reoff\" -> -885714.285714285447   ,  \"Imoff\" -> 0.000000000000   ,  \"στ1\" -> 0.006664321445   ,  \"στS\" -> 0.000168480211   ,  \"στN\" -> 0.000061133182    |>   , \n\"IDS0619_220610_RAW_cal__sam_\" ->   <|    \"ζ\" -> 0.000000000000   ,  \"τ1\" -> 0.000000000000   ,  \"τS\" -> 0.000000000000   ,  \"τN\" -> 0.000000000000   ,  \"τC\" -> 0.000000000000   ,  \"κ0\" -> 0.000000000000   ,  \"mm1\" -> 0.000000000000   ,  \"mm2\" -> 0.000000000000   ,  \"mm3\" -> 0.000000000000   ,  \"T\" -> 1.120000000000   ,  \"B\" -> 8.000000000000   ,  \"θ\" -> 90.000000000000   ,  \"Reoff\" -> 0.000000000000   ,  \"Imoff\" -> 0.000000000000   ,  \"στ1\" -> 0.000000000000   ,  \"στS\" -> 0.000000000000   ,  \"στN\" -> 0.000000000000    |>   , \n\"IDS0620_220610_RAW_cal__ref_\" ->   <|    \"ζ\" -> 0.017708509932   ,  \"τ1\" -> 0.018998736540   ,  \"τS\" -> 0.013522892780   ,  \"τN\" -> 0.000111412007   ,  \"τC\" -> 0.002986591079   ,  \"κ0\" -> 0.000000012545   ,  \"mm1\" -> 0.000042810446   ,  \"mm2\" -> 0.016081465537   ,  \"mm3\" -> 0.019736799645   ,  \"T\" -> 1.900000000000   ,  \"B\" -> 8.000000000000   ,  \"θ\" -> 90.000000000000   ,  \"Reoff\" -> -322448.979591836221   ,  \"Imoff\" -> 0.000000000000   ,  \"στ1\" -> 0.002489183106   ,  \"στS\" -> 0.000085913917   ,  \"στN\" -> 0.000005325276    |>   , \n\"IDS0620_220610_RAW_cal__sam_\" ->   <|    \"ζ\" -> 0.000000000000   ,  \"τ1\" -> 0.000000000000   ,  \"τS\" -> 0.000000000000   ,  \"τN\" -> 0.000000000000   ,  \"τC\" -> 0.000000000000   ,  \"κ0\" -> 0.000000000000   ,  \"mm1\" -> 0.000000000000   ,  \"mm2\" -> 0.000000000000   ,  \"mm3\" -> 0.000000000000   ,  \"T\" -> 1.900000000000   ,  \"B\" -> 8.000000000000   ,  \"θ\" -> 90.000000000000   ,  \"Reoff\" -> 0.000000000000   ,  \"Imoff\" -> 0.000000000000   ,  \"στ1\" -> 0.000000000000   ,  \"στS\" -> 0.000000000000   ,  \"στN\" -> 0.000000000000    |>   , \n\"IDS0621_220610_RAW_cal__ref_\" ->   <|    \"ζ\" -> 0.017222795450   ,  \"τ1\" -> 0.018997433498   ,  \"τS\" -> 0.009525458339   ,  \"τN\" -> 0.000054927338   ,  \"τC\" -> 0.002829107724   ,  \"κ0\" -> 0.000000022378   ,  \"mm1\" -> 0.000037185478   ,  \"mm2\" -> 0.012377068502   ,  \"mm3\" -> 0.019157673942   ,  \"T\" -> 3.100000000000   ,  \"B\" -> 8.000000000000   ,  \"θ\" -> 90.000000000000   ,  \"Reoff\" -> -175510.204081632662   ,  \"Imoff\" -> 0.000000000000   ,  \"στ1\" -> 0.000696462866   ,  \"στS\" -> 0.000049011590   ,  \"στN\" -> 0.000001187946    |>   , \n\"IDS0621_220610_RAW_cal__sam_\" ->   <|    \"ζ\" -> 0.000000000000   ,  \"τ1\" -> 0.000000000000   ,  \"τS\" -> 0.000000000000   ,  \"τN\" -> 0.000000000000   ,  \"τC\" -> 0.000000000000   ,  \"κ0\" -> 0.000000000000   ,  \"mm1\" -> 0.000000000000   ,  \"mm2\" -> 0.000000000000   ,  \"mm3\" -> 0.000000000000   ,  \"T\" -> 3.100000000000   ,  \"B\" -> 8.000000000000   ,  \"θ\" -> 90.000000000000   ,  \"Reoff\" -> 0.000000000000   ,  \"Imoff\" -> 0.000000000000   ,  \"στ1\" -> 0.000000000000   ,  \"στS\" -> 0.000000000000   ,  \"στN\" -> 0.000000000000    |>   , \n\"IDS0622_220610_RAW_cal__ref_\" ->   <|    \"ζ\" -> 0.018802685442   ,  \"τ1\" -> 0.018950322094   ,  \"τS\" -> 0.005932159284   ,  \"τN\" -> 0.000034155015   ,  \"τC\" -> 0.002206206702   ,  \"κ0\" -> 0.000000055128   ,  \"mm1\" -> 0.000029936955   ,  \"mm2\" -> 0.008193499351   ,  \"mm3\" -> 0.019011589520   ,  \"T\" -> 5.700000000000   ,  \"B\" -> 8.000000000000   ,  \"θ\" -> 90.000000000000   ,  \"Reoff\" -> -102040.816326530650   ,  \"Imoff\" -> 0.000000000000   ,  \"στ1\" -> 0.004091041448   ,  \"στS\" -> 0.000125318549   ,  \"στN\" -> 0.000002772070    |>   , \n\"IDS0622_220610_RAW_cal__sam_\" ->   <|    \"ζ\" -> 0.000000000000   ,  \"τ1\" -> 0.000000000000   ,  \"τS\" -> 0.000000000000   ,  \"τN\" -> 0.000000000000   ,  \"τC\" -> 0.000000000000   ,  \"κ0\" -> 0.000000000000   ,  \"mm1\" -> 0.000000000000   ,  \"mm2\" -> 0.000000000000   ,  \"mm3\" -> 0.000000000000   ,  \"T\" -> 5.700000000000   ,  \"B\" -> 8.000000000000   ,  \"θ\" -> 90.000000000000   ,  \"Reoff\" -> 0.000000000000   ,  \"Imoff\" -> 0.000000000000   ,  \"στ1\" -> 0.000000000000   ,  \"στS\" -> 0.000000000000   ,  \"στN\" -> 0.000000000000    |>   , \n\"IDS0624_220611_RAW_cal__ref_\" ->   <|    \"ζ\" -> 0.244976366635   ,  \"τ1\" -> 0.050051466083   ,  \"τS\" -> 0.039788798904   ,  \"τN\" -> 0.065150870551   ,  \"τC\" -> 0.000822741325   ,  \"κ0\" -> 0.000000000926   ,  \"mm1\" -> 0.000159743083   ,  \"mm2\" -> 0.015114289281   ,  \"mm3\" -> 0.166247583438   ,  \"T\" -> 0.200000000000   ,  \"B\" -> 10.000000000000   ,  \"θ\" -> 90.000000000000   ,  \"Reoff\" -> -42285714.285714268700   ,  \"Imoff\" -> 0.000000000000   ,  \"στ1\" -> 0.005729614410   ,  \"στS\" -> 0.001369922504   ,  \"στN\" -> 0.004796157705    |>   , \n\"IDS0624_220611_RAW_cal__sam_\" ->   <|    \"ζ\" -> 0.000000000000   ,  \"τ1\" -> 0.000000000000   ,  \"τS\" -> 0.000000000000   ,  \"τN\" -> 0.000000000000   ,  \"τC\" -> 0.000000000000   ,  \"κ0\" -> 0.000000000000   ,  \"mm1\" -> 0.000000000000   ,  \"mm2\" -> 0.000000000000   ,  \"mm3\" -> 0.000000000000   ,  \"T\" -> 0.200000000000   ,  \"B\" -> 10.000000000000   ,  \"θ\" -> 90.000000000000   ,  \"Reoff\" -> 0.000000000000   ,  \"Imoff\" -> 0.000000000000   ,  \"στ1\" -> 0.000000000000   ,  \"στS\" -> 0.000000000000   ,  \"στN\" -> 0.000000000000    |>   , \n\"IDS0625_220611_RAW_cal__ref_\" ->   <|    \"ζ\" -> 0.341296227559   ,  \"τ1\" -> 0.058698913640   ,  \"τS\" -> 0.044841481218   ,  \"τN\" -> 0.116701971458   ,  \"τC\" -> 0.000719554078   ,  \"κ0\" -> 0.000000000751   ,  \"mm1\" -> 0.000181455745   ,  \"mm2\" -> 0.013579301426   ,  \"mm3\" -> 0.262335334208   ,  \"T\" -> 0.170000000000   ,  \"B\" -> 10.000000000000   ,  \"θ\" -> 90.000000000000   ,  \"Reoff\" -> -78285714.285714283600   ,  \"Imoff\" -> 0.000000000000   ,  \"στ1\" -> 0.006389429330   ,  \"στS\" -> 0.001939647043   ,  \"στN\" -> 0.008335030843    |>   , \n\"IDS0625_220611_RAW_cal__sam_\" ->   <|    \"ζ\" -> 0.000000000000   ,  \"τ1\" -> 0.000000000000   ,  \"τS\" -> 0.000000000000   ,  \"τN\" -> 0.000000000000   ,  \"τC\" -> 0.000000000000   ,  \"κ0\" -> 0.000000000000   ,  \"mm1\" -> 0.000000000000   ,  \"mm2\" -> 0.000000000000   ,  \"mm3\" -> 0.000000000000   ,  \"T\" -> 0.170000000000   ,  \"B\" -> 10.000000000000   ,  \"θ\" -> 90.000000000000   ,  \"Reoff\" -> 0.000000000000   ,  \"Imoff\" -> 0.000000000000   ,  \"στ1\" -> 0.000000000000   ,  \"στS\" -> 0.000000000000   ,  \"στN\" -> 0.000000000000    |>   , \n\"IDS0626_220611_RAW_cal__ref_\" ->   <|    \"ζ\" -> 0.430834214152   ,  \"τ1\" -> 0.067490603382   ,  \"τS\" -> 0.050638360024   ,  \"τN\" -> 0.198477935722   ,  \"τC\" -> 0.000694762859   ,  \"κ0\" -> 0.000000000624   ,  \"mm1\" -> 0.000207784316   ,  \"mm2\" -> 0.011935695755   ,  \"mm3\" -> 0.412486005426   ,  \"T\" -> 0.150000000000   ,  \"B\" -> 10.000000000000   ,  \"θ\" -> 90.000000000000   ,  \"Reoff\" -> -115142857.142857134000   ,  \"Imoff\" -> 0.000000000000   ,  \"στ1\" -> 0.010786487534   ,  \"στS\" -> 0.003944576197   ,  \"στN\" -> 0.021401274735    |>   , \n\"IDS0626_220611_RAW_cal__sam_\" ->   <|    \"ζ\" -> 0.000000000000   ,  \"τ1\" -> 0.000000000000   ,  \"τS\" -> 0.000000000000   ,  \"τN\" -> 0.000000000000   ,  \"τC\" -> 0.000000000000   ,  \"κ0\" -> 0.000000000000   ,  \"mm1\" -> 0.000000000000   ,  \"mm2\" -> 0.000000000000   ,  \"mm3\" -> 0.000000000000   ,  \"T\" -> 0.150000000000   ,  \"B\" -> 10.000000000000   ,  \"θ\" -> 90.000000000000   ,  \"Reoff\" -> 0.000000000000   ,  \"Imoff\" -> 0.000000000000   ,  \"στ1\" -> 0.000000000000   ,  \"στS\" -> 0.000000000000   ,  \"στN\" -> 0.000000000000    |>   , \n\"IDS0627_220611_RAW_cal__ref_\" ->   <|    \"ζ\" -> 0.645741447314   ,  \"τ1\" -> 0.078535889200   ,  \"τS\" -> 0.057272545240   ,  \"τN\" -> 0.457037230896   ,  \"τC\" -> 0.000630659614   ,  \"κ0\" -> 0.000000000513   ,  \"mm1\" -> 0.000246422200   ,  \"mm2\" -> 0.008104140921   ,  \"mm3\" -> 0.917236901039   ,  \"T\" -> 0.120000000000   ,  \"B\" -> 10.000000000000   ,  \"θ\" -> 90.000000000000   ,  \"Reoff\" -> -140857142.857142866000   ,  \"Imoff\" -> 0.000000000000   ,  \"στ1\" -> 0.116986349472   ,  \"στS\" -> 0.055522403404   ,  \"στN\" -> 0.466381863920    |>   , \n\"IDS0627_220611_RAW_cal__sam_\" ->   <|    \"ζ\" -> 0.000000000000   ,  \"τ1\" -> 0.000000000000   ,  \"τS\" -> 0.000000000000   ,  \"τN\" -> 0.000000000000   ,  \"τC\" -> 0.000000000000   ,  \"κ0\" -> 0.000000000000   ,  \"mm1\" -> 0.000000000000   ,  \"mm2\" -> 0.000000000000   ,  \"mm3\" -> 0.000000000000   ,  \"T\" -> 0.120000000000   ,  \"B\" -> 10.000000000000   ,  \"θ\" -> 90.000000000000   ,  \"Reoff\" -> 0.000000000000   ,  \"Imoff\" -> 0.000000000000   ,  \"στ1\" -> 0.000000000000   ,  \"στS\" -> 0.000000000000   ,  \"στN\" -> 0.000000000000    |>   , \n\"IDS0628_220611_RAW_cal__ref_\" ->   <|    \"ζ\" -> 0.162802155917   ,  \"τ1\" -> 0.037674171056   ,  \"τS\" -> 0.033369422942   ,  \"τN\" -> 0.027695234809   ,  \"τC\" -> 0.000875515442   ,  \"κ0\" -> 0.000000001247   ,  \"mm1\" -> 0.000120233008   ,  \"mm2\" -> 0.015940588681   ,  \"mm3\" -> 0.093494980492   ,  \"T\" -> 0.250000000000   ,  \"B\" -> 10.000000000000   ,  \"θ\" -> 90.000000000000   ,  \"Reoff\" -> -23795918.367346938700   ,  \"Imoff\" -> 0.000000000000   ,  \"στ1\" -> 0.002046377961   ,  \"στS\" -> 0.000349741229   ,  \"στN\" -> 0.000860381660    |>   , \n\"IDS0628_220611_RAW_cal__sam_\" ->   <|    \"ζ\" -> 0.000000000000   ,  \"τ1\" -> 0.000000000000   ,  \"τS\" -> 0.000000000000   ,  \"τN\" -> 0.000000000000   ,  \"τC\" -> 0.000000000000   ,  \"κ0\" -> 0.000000000000   ,  \"mm1\" -> 0.000000000000   ,  \"mm2\" -> 0.000000000000   ,  \"mm3\" -> 0.000000000000   ,  \"T\" -> 0.250000000000   ,  \"B\" -> 10.000000000000   ,  \"θ\" -> 90.000000000000   ,  \"Reoff\" -> 0.000000000000   ,  \"Imoff\" -> 0.000000000000   ,  \"στ1\" -> 0.000000000000   ,  \"στS\" -> 0.000000000000   ,  \"στN\" -> 0.000000000000    |>   , \n\"IDS0629_220611_RAW_cal__ref_\" ->   <|    \"ζ\" -> 0.112190833427   ,  \"τ1\" -> 0.032183235509   ,  \"τS\" -> 0.030112114218   ,  \"τN\" -> 0.014171616737   ,  \"τC\" -> 0.000992984849   ,  \"κ0\" -> 0.000000001590   ,  \"mm1\" -> 0.000097554049   ,  \"mm2\" -> 0.016918790619   ,  \"mm3\" -> 0.065411835329   ,  \"T\" -> 0.300000000000   ,  \"B\" -> 10.000000000000   ,  \"θ\" -> 90.000000000000   ,  \"Reoff\" -> -13020408.163265310200   ,  \"Imoff\" -> 0.000000000000   ,  \"στ1\" -> 0.001718489505   ,  \"στS\" -> 0.000227881691   ,  \"στN\" -> 0.000458996023    |>   , \n\"IDS0629_220611_RAW_cal__sam_\" ->   <|    \"ζ\" -> 0.000000000000   ,  \"
